vi "fgv_AOL_Globals.vi"(8 "error in (no error)":errorcluster, 10 "AOL_Globals":T1={"Imaging Protocol"=enum."AOL Z-Stack", "Number of POI"=0, "Number of Miniscans"=0, "Number of Trials"=0, "Number of Cycles "=0, "# Averaged Frames"=0, "Laser power (%)"=0, "Pockels (V)"=0.0, "Acquisition Length (sec)"=0.0, "Fill time (us)"=0.0, "POI Dwell time (us)"=0.0, "Miniscan Dwell time per pixel (us)"=0.0, "PMT 1"=0.0, "PMT 2"=0.0, "Back Apperture (mA)"=200.0, "Frame Size"=200, "Center Frequency"=0.0, "Field of View (um)"=175.0, "Field of View (norm)"=0.0, "DwellTime (us)"=0.0, "Ref Dwell Time (us)"=0.0, "Wavelength (nm)"=0.0, "Zoom"=0.0, "AOL Z"=0.0, "AOL Mode"=enum."Raster", "GridXY"=0.0, "GridZ"=0.0, "TriggerPeriod (sec)"=0.0, "Number of Pixels in Miniscan"=0, "Experiment folder path"=path "", "X centre"=0.0, "Y centre"=0.0, "Angle (degrees)"=0.0, "Angle Xs (degrees)"=0.0, "Angle Ys (degrees)"=0.0, "Plane Mode"=0, "Threshold"=[], "Regenerate Chirps"=FALSE, "Rectangle ROI length (pixels)"=0, "Rectangle ROI height (pixels)"=0, "AOD fill"=4900, "StartupDelay"=0, "Samples Wait after Trigger"=5080, "Slip Cycle"=600000, "Add Cycle"=TRUE, "Functional Mode"=enum."Point", "Z Start"=0.0, "Z Stop"=0.0, "# Planes"=0, "Total Pixels"=0, "Variable Miniscan Pixels"=[], "Use Variable Length"=FALSE, "Use Variable Resolution"=FALSE, "Laser power (%) at Z Start"=0, "Laser power (%) at Z Stop"=0, "Ref Z Step"=0} {"Angle Ys (degrees)" format="%#.6g"; "Angle Xs (degrees)" format="%#.6g"; "Plane Mode" items=["XY Plane", "XZ Plane", "YZ Plane", "arbitraryplane"]; "Frame Size" items=["100X100"=100, "128X128"=128, "200X200"=200, "256X256"=256, "512X512"=512, "1024x1024"=1024, "2048x2048"=2048]; "Back Apperture (mA)" format="%#.6g"; "Pockels (V)" format="%#.6g"; "PMT 2" format="%#.6g"; "PMT 1" format="%#.6g"; "Angle (degrees)" format="%#.6g"; "POI Dwell time (us)" format="%#.6g"}, 11 "Function":enum16{"Intialize", "Write", "Read", "Clear"}(ring)) -> (0 "error out":errorcluster, 2 "AOL_Globals":T1={"Imaging Protocol"=enum."AOL Z-Stack", "Number of POI"=0, "Number of Miniscans"=0, "Number of Trials"=0, "Number of Cycles "=0, "# Averaged Frames"=0, "Laser power (%)"=0, "Pockels (V)"=0.0, "Acquisition Length (sec)"=0.0, "Fill time (us)"=0.0, "POI Dwell time (us)"=0.0, "Miniscan Dwell time per pixel (us)"=0.0, "PMT 1"=0.0, "PMT 2"=0.0, "Back Apperture (mA)"=0.0, "Frame Size"=200, "Center Frequency"=0.0, "Field of View (um)"=175.0, "Field of View (norm)"=0.0, "DwellTime (us)"=0.0, "Ref Dwell Time (us)"=0.0, "Wavelength (nm)"=0.0, "Zoom"=0.0, "AOL Z"=0.0, "AOL Mode"=enum."Raster", "GridXY"=0.0, "GridZ"=0.0, "TriggerPeriod (sec)"=0.0, "Number of Pixels in Miniscan"=0, "Experiment folder path"=path "", "X centre"=0.0, "Y centre"=0.0, "Angle (degrees)"=0.0, "Angle Xs (degrees)"=0.0, "Angle Ys (degrees)"=0.0, "Plane Mode"=0, "Threshold"=[], "Regenerate Chirps"=FALSE, "Rectangle ROI length (pixels)"=0, "Rectangle ROI height (pixels)"=0, "AOD fill"=4900, "StartupDelay"=0, "Samples Wait after Trigger"=5080, "Slip Cycle"=600000, "Add Cycle"=TRUE, "Functional Mode"=enum."Point", "Z Start"=0.0, "Z Stop"=0.0, "# Planes"=0, "Total Pixels"=0, "Variable Miniscan Pixels"=[], "Use Variable Length"=FALSE, "Use Variable Resolution"=FALSE, "Laser power (%) at Z Start"=0, "Laser power (%) at Z Stop"=0, "Ref Z Step"=0} {"Angle Ys (degrees)" format="%#.6g"; "Angle Xs (degrees)" format="%#.6g"; "Plane Mode" items=["XY Plane", "XZ Plane", "YZ Plane", "arbitraryplane"]; "Frame Size" items=["100X100"=100, "128X128"=128, "200X200"=200, "256X256"=256, "512X512"=512, "1024x1024"=1024, "2048x2048"=2048]; "Back Apperture (mA)" format="%#.6g"; "Pockels (V)" format="%#.6g"; "PMT 2" format="%#.6g"; "PMT 1" format="%#.6g"; "Angle (degrees)" format="%#.6g"; "POI Dwell time (us)" format="%#.6g"})   [LabVIEW 2020]
uses:
  Typedefs/Controls/AOL_Globals.ctl
  Typedefs/Imaging Protocols enum.ctl
  Typedefs/Frame Size.ctl
  Typedefs/AOL modes.ctl
  Typedefs/Plane Mode.ctl
  Typedefs/Functional Mode.ctl
  General Globals.vi
panel:
  # "WARNING! SET AS SUBROUTINE"
  # "<---- NOTE!  I don't think the PMT1\n          and PMT2 values are used. Elliminate."
  # "<---- NOTE!  I don't think the PMT1\n          and PMT2 values are used. Elliminate."
  # "<---- NOTE!  Normalised FOV value"
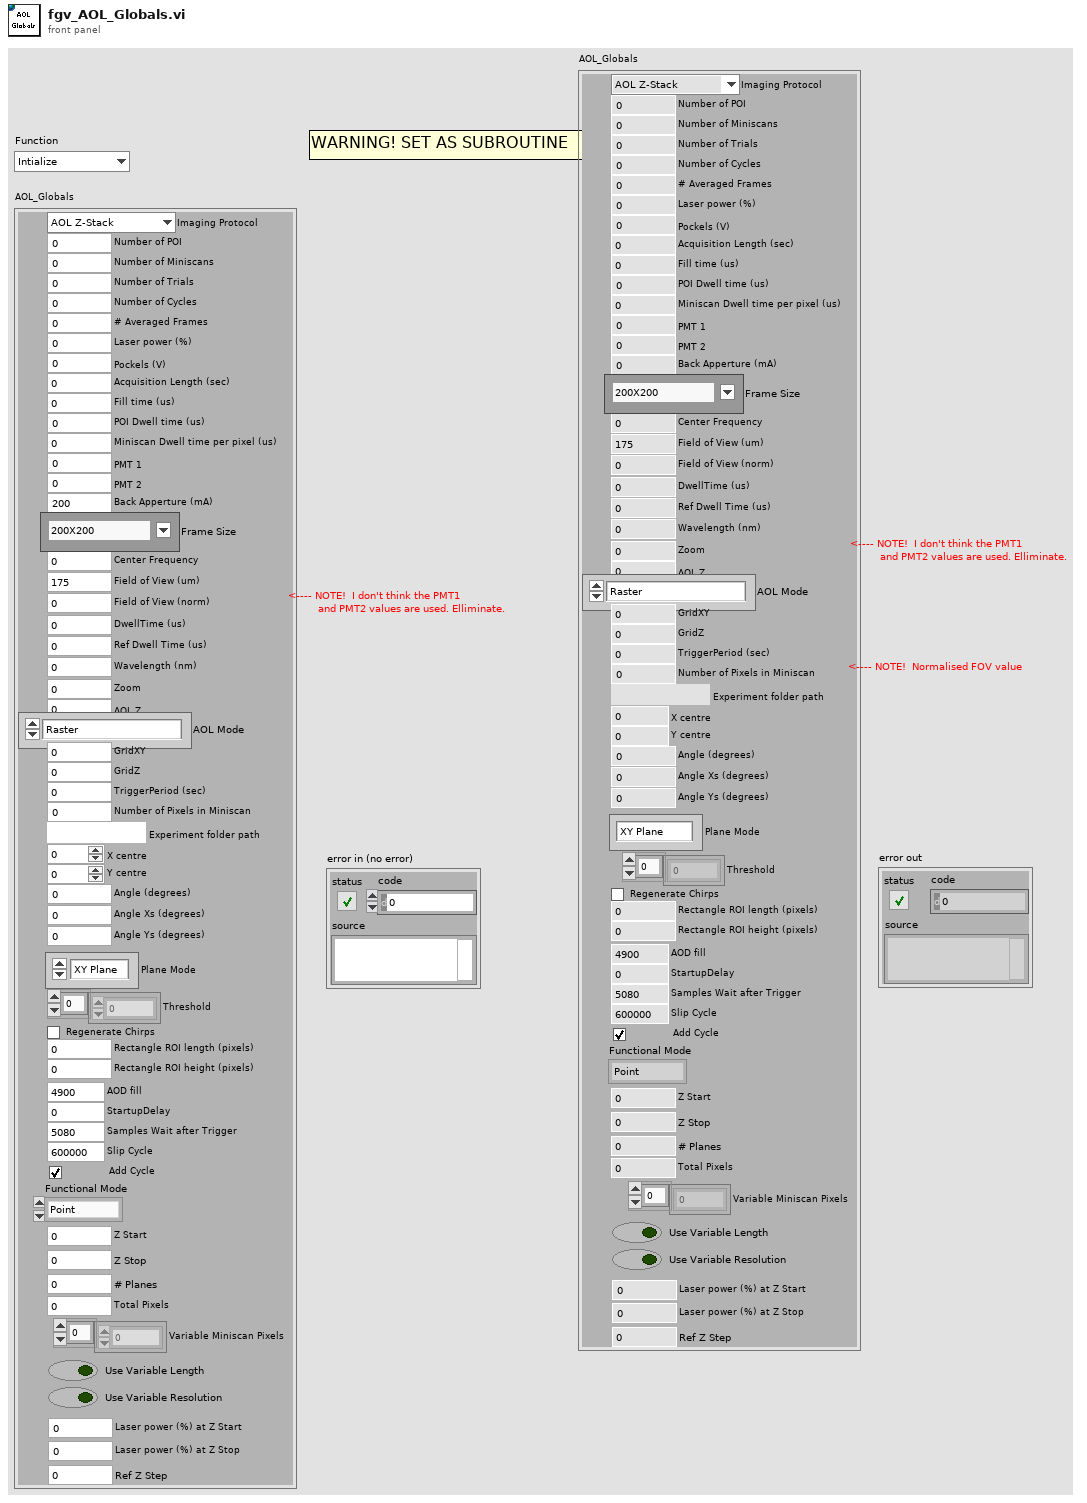
[diagram p1: front panel]
types:
  T1 = typedef "AOL_Globals.ctl" = cluster{"Imaging Protocol":T2, "Number of POI":u16, "Number of Miniscans":u16, "Number of Trials":u16, "Number of Cycles ":u64, "# Averaged Frames":u16, "Laser power (%)":u8, "Pockels (V)":dbl, "Acquisition Length (sec)":dbl, "Fill time (us)":dbl, "POI Dwell time (us)":dbl, "Miniscan Dwell time per pixel (us)":dbl, "PMT 1":dbl, "PMT 2":dbl, "Back Apperture (mA)":dbl, "Frame Size":T3, "Center Frequency":dbl, "Field of View (um)":dbl, "Field of View (norm)":dbl, "DwellTime (us)":dbl, "Ref Dwell Time (us)":dbl, "Wavelength (nm)":dbl, "Zoom":dbl, "AOL Z":dbl, "AOL Mode":T4, "GridXY":dbl, "GridZ":dbl, "TriggerPeriod (sec)":dbl, "Number of Pixels in Miniscan":u16, "Experiment folder path":path, "X centre":dbl, "Y centre":dbl, "Angle (degrees)":dbl, "Angle Xs (degrees)":dbl, "Angle Ys (degrees)":dbl, "Plane Mode":T5, "Threshold":u16[], "Regenerate Chirps":bool, "Rectangle ROI length (pixels)":u16, "Rectangle ROI height (pixels)":u16, "AOD fill":u16, "StartupDelay":i32, "Samples Wait after Trigger":u16, "Slip Cycle":u32, "Add Cycle":bool, "Functional Mode":T6, "Z Start":dbl, "Z Stop":dbl, "# Planes":i32, "Total Pixels":i32, "Variable Miniscan Pixels":u16[], "Use Variable Length":bool, "Use Variable Resolution":bool, "Laser power (%) at Z Start":u8, "Laser power (%) at Z Stop":u8, "Ref Z Step":i8}
  T2 = typedef "Imaging Protocols enum.ctl" = enum16{"AOL Z-Stack", "Motor Z Stack", "Parameter Sweep", "Functional Acquisition", "Single Plane Acquisition", "Volume Acquisition", "Live Imaging", "Live Plane Imaging", "Live Volume Imaging"}
  T3 = typedef "Frame Size.ctl" = u16
  T4 = typedef "AOL modes.ctl" = enum16{"Raster", "Structural", "Pointing", "Mini Scan", "Alignment"}
  T5 = typedef "Plane Mode.ctl" = u16
  T6 = typedef "Functional Mode.ctl" = enum16{"Point", "Line", "Patch", "Plane", "Volume"}
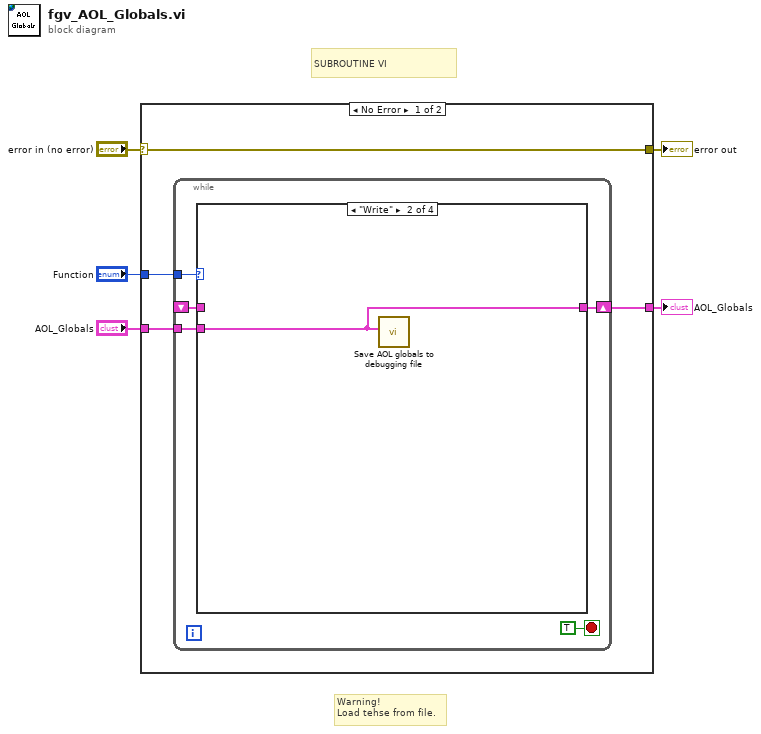
[diagram p0: block diagram]
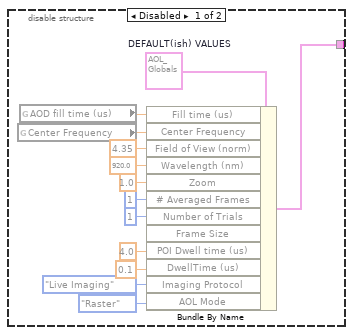
[diagram p3: hidden frame]
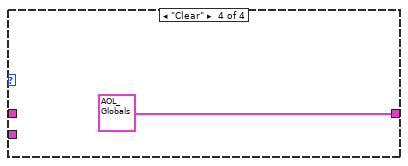
[diagram p5: hidden frame]
diagram:
  # "SUBROUTINE VI"
  # "Warning!\nLoad tehse from file."
  n1 = case shown="No Error" "error in (no error)" {
    selector: "error in (no error)" -> [w6 w34]
    tunnel: [w6 w34] -> w4
    tunnel: "Function" -> [w9 _]
    tunnel: "AOL_Globals" -> [w8 w33]
    tunnel: [w7 w33] -> w1
    frame No Error {
      n2 = while {
        tunnel: w9 -> [w13]
        tunnel: w8 -> [w12]
        shift-right: [w11] -> w7
        shift-left: _ -> [w10]
        stop <- TRUE stop-if-true
        n3 = case shown="\"Write\"" w13 {
          tunnel: [w15 w30 w31 T1 {"Imaging Protocol"=enum."AOL Z-Stack", "Number of POI"=0, "Number of Miniscans"=0, "Number of Trials"=0, "Number of Cycles "=0, "# Averaged Frames"=0, "Laser power (%)"=0, "Pockels (V)"=0.0, "Acquisition Length (sec)"=0.0, "Fill time (us)"=0.0, "POI Dwell time (us)"=0.0, "Miniscan Dwell time per pixel (us)"=0.0, "PMT 1"=0.0, "PMT 2"=0.0, "Back Apperture (mA)"=0.0, "Frame Size"=0, "Center Frequency"=0.0, "Field of View (um)"=175.0, "Field of View (norm)"=0.0, "DwellTime (us)"=0.0, "Ref Dwell Time (us)"=0.0, "Wavelength (nm)"=0.0, "Zoom"=0.0, "AOL Z"=0.0, "AOL Mode"=enum."Raster", "GridXY"=0.0, "GridZ"=0.0, "TriggerPeriod (sec)"=0.0, "Number of Pixels in Miniscan"=0, "Experiment folder path"=path "", "X centre"=0.0, "Y centre"=0.0, "Angle (degrees)"=0.0, "Angle Xs (degrees)"=0.0, "Angle Ys (degrees)"=0.0, "Plane Mode"=0, "Threshold"=[], "Regenerate Chirps"=FALSE, "Rectangle ROI length (pixels)"=0, "Rectangle ROI height (pixels)"=0, "AOD fill"=0, "StartupDelay"=0, "Samples Wait after Trigger"=0, "Slip Cycle"=0, "Add Cycle"=FALSE, "Functional Mode"=enum."Point", "Z Start"=0.0, "Z Stop"=0.0, "# Planes"=0, "Total Pixels"=0, "Variable Miniscan Pixels"=[], "Use Variable Length"=FALSE, "Use Variable Resolution"=FALSE, "Laser power (%) at Z Start"=0, "Laser power (%) at Z Stop"=0, "Ref Z Step"=0} ("AOL_Globals")] -> w11
          tunnel: w12 -> [_ w30 _ _]
          tunnel: w10 -> [_ _ w31 _]
          frame "Intialize", Default {
            # "REDUNDANT CASE. THIS FGV IS NOW INITIALISED FROM FILE BY THE \"Save-Load Initial Values.vi\""
            n4 = disable-structure shown="Enabled" {
              disable-tunnel: [w26 _] -> w15
              frame Disabled {
                w16 = T1 {"Imaging Protocol"=enum."Live Imaging", "Number of POI"=0, "Number of Miniscans"=0, "Number of Trials"=0, "Number of Cycles "=0, "# Averaged Frames"=1, "Laser power (%)"=35, "Pockels (V)"=0.0, "Acquisition Length (sec)"=0.0, "Fill time (us)"=24.4, "POI Dwell time (us)"=0.0, "Miniscan Dwell time per pixel (us)"=0.0, "PMT 1"=0.0, "PMT 2"=0.0, "Back Apperture (mA)"=0.0, "Frame Size"=200, "Center Frequency"=38.0, "Field of View (um)"=175.0, "Field of View (norm)"=4.349999904632568, "DwellTime (us)"=0.10000000149011612, "Ref Dwell Time (us)"=0.0, "Wavelength (nm)"=800.0, "Zoom"=1.0, "AOL Z"=0.0, "AOL Mode"=enum."Raster", "GridXY"=0.0, "GridZ"=0.0, "TriggerPeriod (sec)"=0.0, "Number of Pixels in Miniscan"=0, "Experiment folder path"=path "", "X centre"=0.0, "Y centre"=0.0, "Angle (degrees)"=0.0, "Angle Xs (degrees)"=0.0, "Angle Ys (degrees)"=0.0, "Plane Mode"=0, "Threshold"=[], "Regenerate Chirps"=FALSE, "Rectangle ROI length (pixels)"=0, "Rectangle ROI height (pixels)"=0, "AOD fill"=0, "StartupDelay"=0, "Samples Wait after Trigger"=0, "Slip Cycle"=0, "Add Cycle"=FALSE, "Functional Mode"=enum."Point", "Z Start"=0.0, "Z Stop"=0.0, "# Planes"=0, "Total Pixels"=0, "Variable Miniscan Pixels"=[], "Use Variable Length"=FALSE, "Use Variable Resolution"=FALSE, "Laser power (%) at Z Start"=0, "Laser power (%) at Z Stop"=0, "Ref Z Step"=0}  # DEFAULT(ish) VALUES
                n5 = global read "General Globals.vi" "Center Frequency"() -> (w24:dbl)
                n6 = global read "General Globals.vi" "AOD fill time (us)"() -> (w23:dbl)
                n7 = Bundle By Name(cluster=w16, "Fill time (us)"=w23, "Center Frequency"=w24, "Field of View (norm)"=4.35 ("Field of View"), "Wavelength (nm)"=920.0, "Zoom"=1.0, "# Averaged Frames"=u16 1, "Number of Trials"=u16 1, "POI Dwell time (us)"=4.0, "DwellTime (us)"=0.1, "Imaging Protocol"=Imaging_Protocols_enum."Live Imaging", "AOL Mode"=AOL_modes."Raster") -> (w26:T1, "Frame Size"=w17:T3)
              }
              frame Enabled {
              }
            }
          }
          frame "Write" {
            n8 = call "Save AOL globals to debugging file.vi"("AOL_Globals"=w30) -> ()  [unwired: 11 in]
          }
          frame "Read" {
          }
          frame "Clear" {
          }
        }
      }
    }
    frame Error {
    }
  }
  "error out" <- w4
  "AOL_Globals" <- w1
